vi "Make new Filename.vi"(6 "Filetype (default=.png)":string, 7 "Read only?(F)":bool, 8 "error in (no error)":errorcluster, 10 "start path":path, 11 "Must prompt for path? (F)":bool) -> (0 "error out":errorcluster, 1 "File #":i32, 2 "Scan Filepath":path, 3 "Cancelled?":bool, 4 "Base file":path)   [LabVIEW 2013]
doc: "This is a functional global that produces an autoincrementing filename. On first call or if specified, the .vi will prompt the user for a base filename."
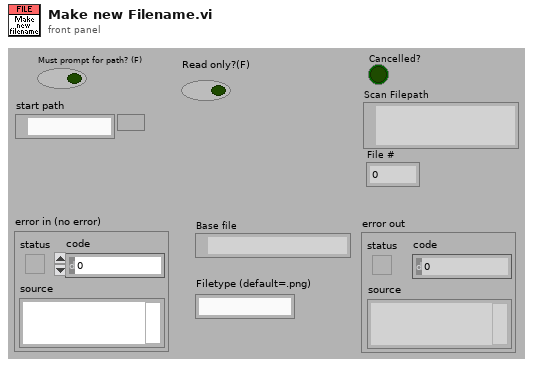
[diagram p1: front panel]
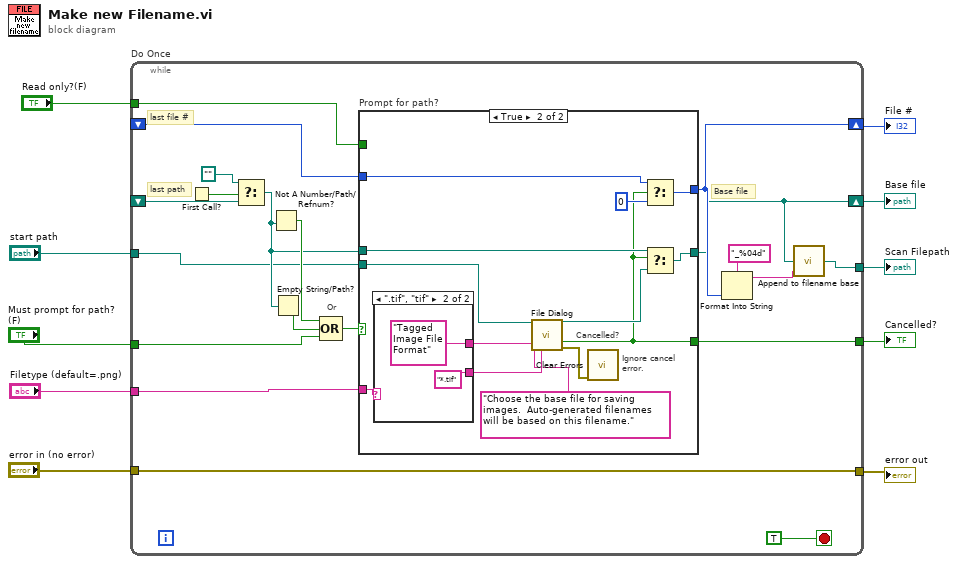
[diagram p0: block diagram]
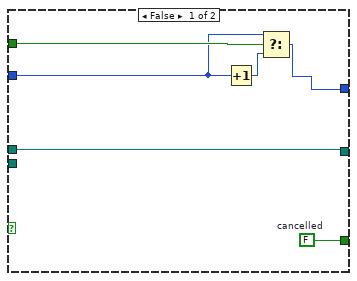
[diagram p2: hidden frame]
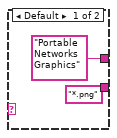
[diagram p3: hidden frame]
diagram:
  n1 = while "Do Once" {
    shift-right: [w23] -> w6
    shift-left: _ -> [w29]
    tunnel: "Must prompt for path? (F)" -> [w24]
    tunnel: [w14] -> w9
    shift-right: [w17] -> w4
    shift-left: _ -> [w21]
    tunnel: [w30] -> w8
    tunnel: "error in (no error)" -> [w14]
    tunnel: [w15] -> w5
    tunnel: "Filetype (default=.png)" -> [w13]
    tunnel: "start path" -> [w12]
    tunnel: "Read only?(F)" -> [w11]
    stop <- TRUE stop-if-true
    # "last path"
    # "Or"
    # "Base file"
    # "last file #"
    n2 = First Call?() -> (First Call?: T/F=w19:bool)
    n3 = Select(t=path "", s=w19, f=w21) -> (s? t:f=w20:path)
    n4 = Not A Number/Path/Refnum?(number/path/refnum=w20) -> (NaN/Path/Refnum?=w25:bool)
    n5 = Empty String/Path?(string/path=w20) -> (empty?=w26:bool)
    n6 = Compound Arithmetic op=OR(w25, w26, w24) -> (w27:bool)
    n7 = case "Prompt for path?" shown="True" w27 {
      tunnel: [w36 w42] -> w30
      tunnel: w29 -> [w33 w48]
      tunnel: [w31 w47] -> w23
      tunnel: [w35 w44] -> w17
      tunnel: w20 -> [w35 w45]
      tunnel: w13 -> [_ w38]
      tunnel: w12 -> [_ w37]
      tunnel: w11 -> [w34 _]
      frame False {
        w36 = FALSE  # cancelled
        n8 = Increment(x=w33) -> (x+1=w32:i32)
        n9 = Select(t=w33, s=w34, f=w32) -> (s? t:f=w31:i32)
      }
      frame True {
        # "Ignore cancel\nerror."
        # "Cancelled?"
        n10 = case shown="\".tif\", \"tif\"" w38 {
          tunnel: ["*.png" ("pattern (all files)") "*.tif" ("pattern (all files)")] -> w49
          tunnel: ["Portable Networks Graphics" ("pattern label") "Tagged Image File Format" ("pattern label")] -> w39
          frame Default {
          }
          frame ".tif", "tif" {
          }
        }
        n11 = call "File Dialog"("start path"=w37, "prompt"="Choose the base file for saving images.  Auto-generated filenames will be based on this filename.", "pattern (all files)"=w49, "pattern label"=w39) -> ("selected path"=w43:path, "cancelled"=w42:bool, "error out"=w41:errorcluster)  [unwired: 3 in, 6 out]
        n12 = call <vilib>:"Clear Errors.vi"("error in (no error)"=w41) -> ()  [unwired: 7 out]
        n13 = Select(t=w48, s=w42, f=0) -> (s? t:f=w47:i32)
        n14 = Select(t=w45, s=w42, f=w43) -> (s? t:f=w44:path)
      }
    }
    n15 = Format Into String(format string="_%04d", w23) -> (resulting string=w16:string)  [unwired: 2 in, 1 out]
    n16 = call "Append to filename base.vi"("Text to append to base"=w16, "Path"=w17) -> ("Path out"=w15:path)  [unwired: 3 out]
  }
  "File #" <- w6
  "error out" <- w9
  "Scan Filepath" <- w5
  "Cancelled?" <- w8
  "Base file" <- w4
